vi "ORS_LinearizeFringe-CallDLL.vi"(7 "path in":path=path "\\\\Johann\\ag-huber/Programs/Imaging/C/wwimgdll64/wwimgdll/Release-x64/wwimgdll.dll", 9 "method":i32, 10 "Ch1 Michelson":dbl[](array[numeric]), 11 "Hilbert in":dbl[](array[numeric]) caption="inverted Hilbert in") -> (0 "error count":i32, 1 "error out":errorcluster, 3 "Ch1 linearized":dbl[](array[numeric]) format="%_6g")   [LabVIEW 2016]
uses:
  <vilib>/Utility/error.llb/DialogType.ctl
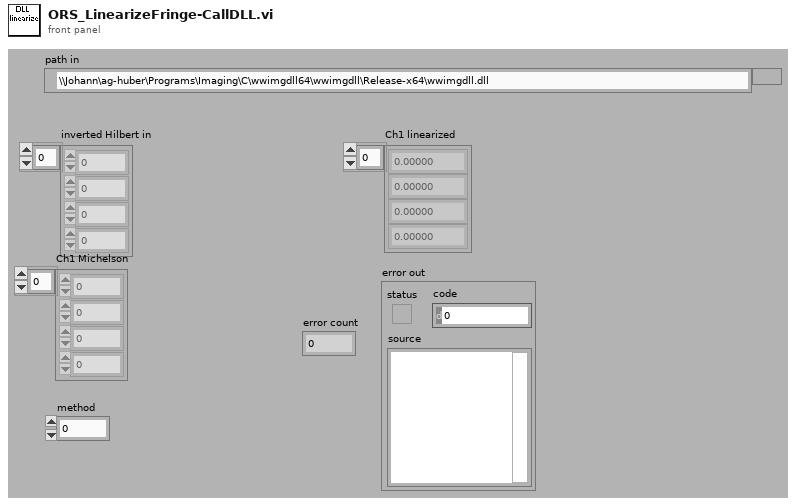
[diagram p1: front panel]
types:
  T1 = typedef "DialogType.ctl" = u16
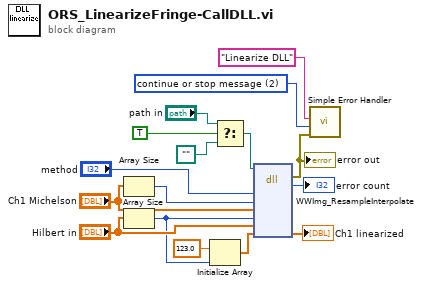
[diagram p0: block diagram]
diagram:
  w1 = T1 2 items=["no dialog", "OK message", "continue or stop message", "OK message + warnings", "continue/stop + warnings"] ("type of dialog (OK msg:1)")
  n1 = Array Size(array="Ch1 Michelson") -> (size(s)=w8:i32)
  n2 = Array Size(array="Hilbert in") -> (size(s)=w3:i32)
  n3 = Initialize Array(123.0 ("element"), w3) -> (w5:dbl[])
  n4 = Select(t="path in", s=TRUE, f=path "") -> (s? t:f=w15:path)
  n5 = dll-call lib="\\\\Johann\\ag-huber/Programs/Imaging/C/wwimgdll64/wwimgdll/Release-x64/wwimgdll.dll" fn="WWImg_ResampleInterpolate" ("ww_interpolate.dll:?testdll@@YAXHPAN0@Z")(path in=w15, "method"="method", "ndata"=w8, "data"="Ch1 Michelson", "ninterp"=w3, "xvals"="Hilbert in", "iout"=w5) -> (error out=w11:errorcluster, "return type"=→"error count":i32, "iout"=→"Ch1 linearized":dbl[])  [unwired: 7 in, 1 out]
  "error out" <- w11
  n6 = call <vilib>:"Simple Error Handler.vi"("error source (\" \")"="Linearize DLL" ("error source (\" \")"), "type of dialog (OK msg:1)"=w1, "error in (no error)"=w11) -> ()  [unwired: 2 in, 5 out]
